vi "Reset Buffer.vi"(8 "error in (no error)":errorcluster, 11 "DeviceRefnum":u64) -> (0 "error out":errorcluster, 2 "function return":i32, 3 "DeviceRefnum Out":u64)   [LabVIEW 2014]
doc: "Resets the streaming buffer."
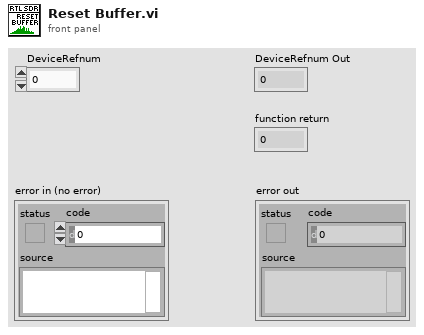
[diagram p1: front panel]
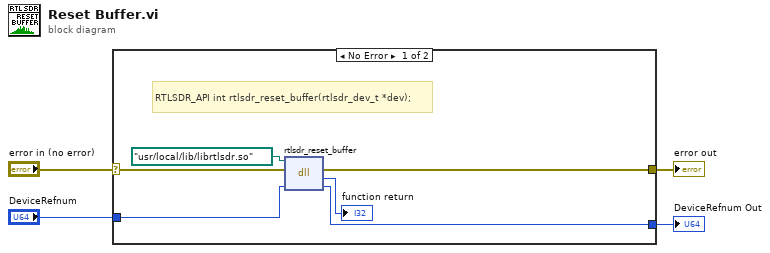
[diagram p0: block diagram]
diagram:
  n1 = case shown="No Error" "error in (no error)" {
    selector: "error in (no error)" -> [w5 w11]
    tunnel: [w9 w11] -> w4
    tunnel: "DeviceRefnum" -> [w8 w12]
    tunnel: [w7 w12] -> w2
    frame No Error {
      # "RTLSDR_API int rtlsdr_reset_buffer(rtlsdr_dev_t *dev);"
      n2 = dll-call lib="C:/Program Files (x86)/National Instruments/LabVIEW 2016/user.lib/rtlsdr/rtlsdr.*" fn="rtlsdr_reset_buffer"(path in=path "/usr/local/lib/librtlsdr.so", error in=w5, "DeviceRefnum"=w8) -> (error out=w9:errorcluster, "return type"=→"function return":i32, "DeviceRefnum"=w7:u64)  [unwired: 1 in, 1 out]
    }
    frame Error {
    }
  }
  "error out" <- w4
  "DeviceRefnum Out" <- w2
